vi "Sort Weekly Data (SubVI).vi"(8 "error in (no error)":errorcluster, 11 "Data Value Reference in":refnum<data-value>) -> (0 "error out":errorcluster, 3 "Data Value Reference out":refnum<data-value>)   [LabVIEW 2017, in "DS_Lib.lvlib" / "SRReportParser.lvlib"]
uses:
  SRReportParser.lvlib
  TypeDefs/WeeklyData.ctl
  Modules/Private Controls/Data Raw.ctl
  Modules/Private Controls/Report Data Cluster.ctl
  Modules/Data Operations.lvlib
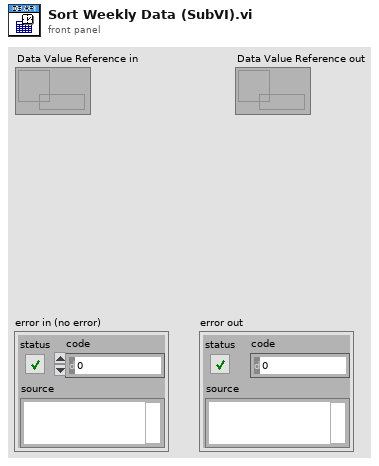
[diagram p1: front panel]
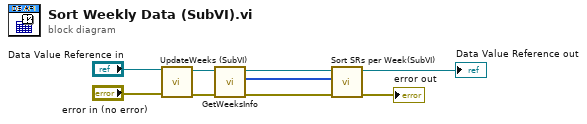
[diagram p0: block diagram]
diagram:
  n1 = call "UpdateWeeks (SubVI).vi"("Error In"="error in (no error)", "DVR In"="Data Value Reference in") -> ("Error Out"=w6:errorcluster, "DVR Out"=w5:refnum<data-value>)  [unwired: 8 in]
  n2 = call "GetWeeksInfo.vi"("error in (no error)"=w6, "Data Value Reference in"=w5) -> ("error out"=w2:errorcluster, "List of Weeks"=w7:u8[], "Data Value Reference out"=w1:refnum<data-value>)  [unwired: 7 in]
  n3 = call "Sort SRs per Week(SubVI).vi"("error in (no error)"=w2, "Weeks"=w7, "Data Value Reference in"=w1) -> ("error out"=→"error out":errorcluster, "DVR Weekly/Country Data"=→"Data Value Reference out":refnum<data-value>)  [unwired: 7 in]
